vi "Start Sync.vi"(8 "error in (no error)":errorcluster, 11 "Log Record in":refnum<class "Log Record.lvclass">) -> (0 "error out":errorcluster, 3 "Log Record out":refnum<class "Log Record.lvclass">)   [LabVIEW 2024, in "Log Record.lvclass"]
uses:
  Log Record.lvclass
  C:/Program Files/National Instruments/LabVIEW 2025/vi.lib/ActorFramework/Actor/Actor.lvclass
  Log Record Messages/Get OSF Status Msg/Get OSF Status Msg.lvclass
  C:/Program Files/National Instruments/LabVIEW 2025/vi.lib/ActorFramework/Message/Message.lvclass
  Log Record.lvclass/Log Record.ctl
  <vilib>/ActorFramework/Actor/Actor.lvclass/Actor.ctl
  <vilib>/ActorFramework/Message Enqueuer/Message Enqueuer.lvclass/Message Enqueuer.ctl
  <vilib>/ActorFramework/Message Enqueuer/Message Enqueuer.lvclass
  <vilib>/ActorFramework/Actor Framework.lvlib
  <vilib>/ActorFramework/Actor/Actor.lvclass
  Log Record State.ctl
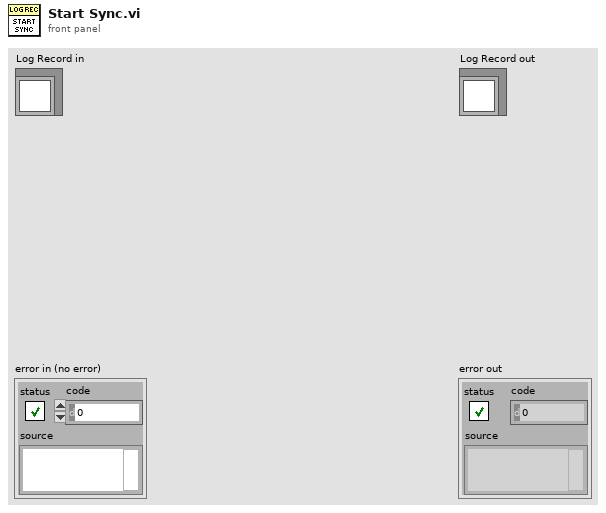
[diagram p1: front panel]
types:
  T1 = typedef "Log Record State.ctl" = enum16{"Idle", "Requested login", "Logged on", "Requested logout", "Logged off"}
  T2 = typedef "Log Record Configuration.ctl" = cluster{"OSF node  ID":string, "Conection timeout":dbl, "Station":string, "Log server ":string, "Upload to OSF":bool, "Append to lab book":bool, "Filing modules":string[], "File prefix":string, "Computer":string}
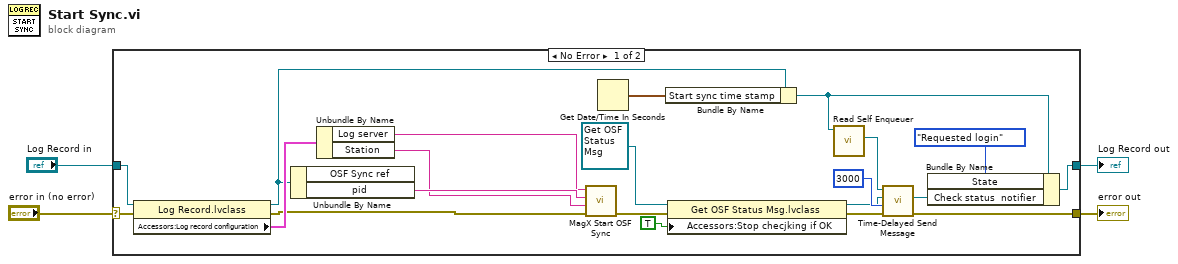
[diagram p0: block diagram]
diagram:
  n1 = case shown="No Error" "error in (no error)" {
    selector: "error in (no error)" -> [w25 w27]
    tunnel: [w16 w27] -> w3
    tunnel: [w15 w26] -> w1
    tunnel: "Log Record in" -> [w23 w26]
    frame No Error {
      n2 = property class="Log Record.lvclass"(reference=w23, error in=w25) -> (reference out=w19:refnum<class "Log Record.lvclass">, error out=w8:errorcluster, "Accessors:Log record configuration"=w22:T2)
      n3 = Unbundle By Name(w19) -> ("pid"=w24:string)  [unwired: 1 out]
      n4 = Unbundle By Name(w22) -> ("Log server"=w20:string, "Station"=w21:string)
      n5 = call "MagX Start OSF Sync.vi"("error in"=w8, "Station"=w21, "Experiment ID"=w24, "MagLab OSF tool server"=w20) -> ("error out"=w17:errorcluster)  [unwired: 7 in]
      n6 = Get Date/Time In Seconds() -> (seconds since 1Jan1904=w6:timestamp)
      n7 = Bundle By Name(cluster=w19, "Start sync time stamp"=w6) -> (w7:refnum<class "Log Record.lvclass">)
      n8 = property class="Get OSF Status Msg.lvclass"(reference=refnum<class "Get OSF Status Msg.lvclass"> refnum ("Get OSF Status Msg.lvclass"), error in=w17, "Accessors:Stop checjking if OK"=TRUE ("Stop checjking if OK")) -> (reference out=w10:refnum<class "Get OSF Status Msg.lvclass">, error out=w12:errorcluster)
      n9 = call <vilib>:"Read Self Enqueuer.vi"("Actor"=w7) -> ("Self Enqueuer"=w18:refnum<class "Message Enqueuer.lvclass">)  [unwired: 10 in]
      n10 = call <vilib>:"Time-Delayed Send Message.vi"("error in (no error)"=w12, "Milliseconds To Wait"=3000, "Message"=w10, "Message Enqueuer"=w18) -> ("error out"=w16:errorcluster, "Delivery Notifier"=w14:refnum<notifier>)  [unwired: 6 in]
      n11 = Bundle By Name(cluster=w7, "State"=Log_Record_State."Requested login", "Check status  notifier"=w14) -> (w15:refnum<class "Log Record.lvclass">)
    }
    frame Error {
    }
  }
  "error out" <- w3
  "Log Record out" <- w1
